vi "WSVCAP SHL Host TL I2C Read - Single Device.vi"(0 "Bytes to Read (1-4)":u8=4 min=1 max=4 step=1, 5 "Sub Address [U8]":u8=191 format="%.0x", 11 "error in":errorcluster, 12 "DUT":T2, 13 "Device":T1, 14 "Log (T)":bool=TRUE) -> (4 "Device Data":u8[](array[numeric]) format="%.0x", 15 "error out":errorcluster)   [LabVIEW 2012]
uses:
  Type Defs/WSVCAP SHL DUT Number Enum.ctl
  Type Defs/WSVCAP SHL I2C Device Enum.ctl
panel:
  out "C3:1-36 Read Data [U8]":u8[][](array[numeric]) format="%.0x"
  out "Socket Mask Set [U64]":u64[](array[numeric]) format="%012x"
  out "C2:1-36 Read Data [U8]":u8[][](array[numeric]) format="%.0x"
  out "C1:1-36 Read Data [U8]":u8[][](array[numeric]) format="%.0x"
  out "Data Headers":u8[](array[numeric])=[1, 2, 3, 4, 5, 6, 7, 8, 9, 10, 11, 12, 12, 14, 15, 16, 17, 18, 19, 20, 21, 22, 23, 24, 25, 26, 27, 28, 29, 30, 31, 32, 33, 34, 35, 36]
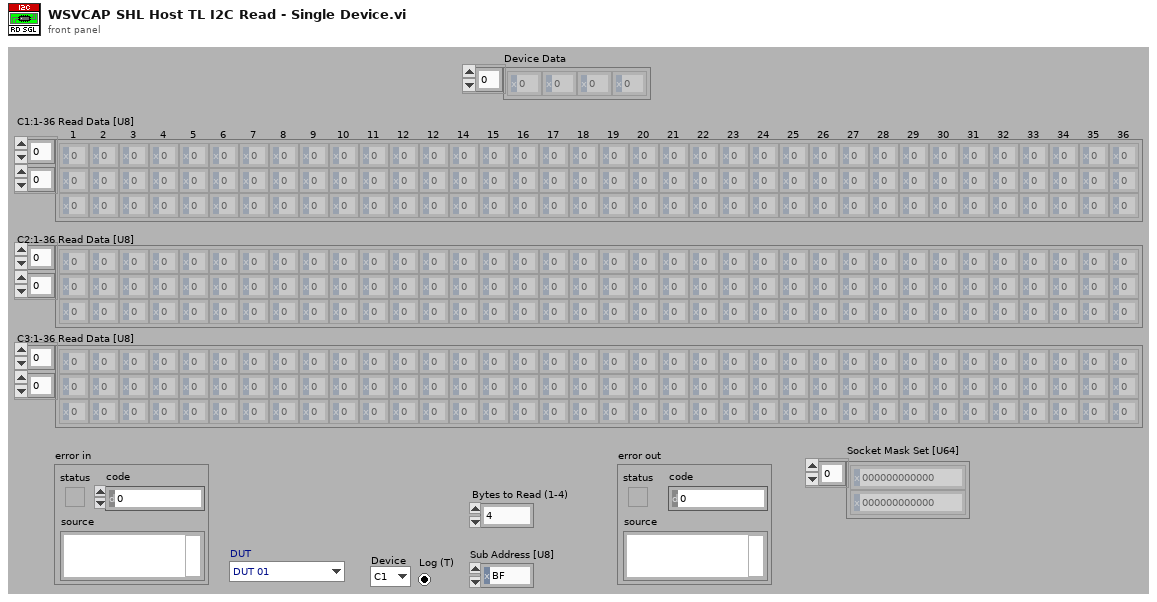
[diagram p1: front panel]
types:
  T1 = typedef "WSVCAP SHL I2C Device Enum.ctl" = enum16{"C1", "C2", "C3"}
  T2 = typedef "WSVCAP SHL DUT Number Enum.ctl" = enum16{"DUT 01", "DUT 02", "DUT 03", "DUT 04", "DUT 05", "DUT 06", "DUT 07", "DUT 08", "DUT 09", "DUT 10", "DUT 11", "DUT 12", "DUT 13", "DUT 14", "DUT 15", "DUT 16", "DUT 17", "DUT 18", "DUT 19", "DUT 20", "DUT 21", "DUT 22", "DUT 23", "DUT 24", "DUT 25", "DUT 26", "DUT 27", "DUT 28", "DUT 29", "DUT 30", "DUT 31", "DUT 32", "DUT 33", "DUT 34", "DUT 35", "DUT 36"}
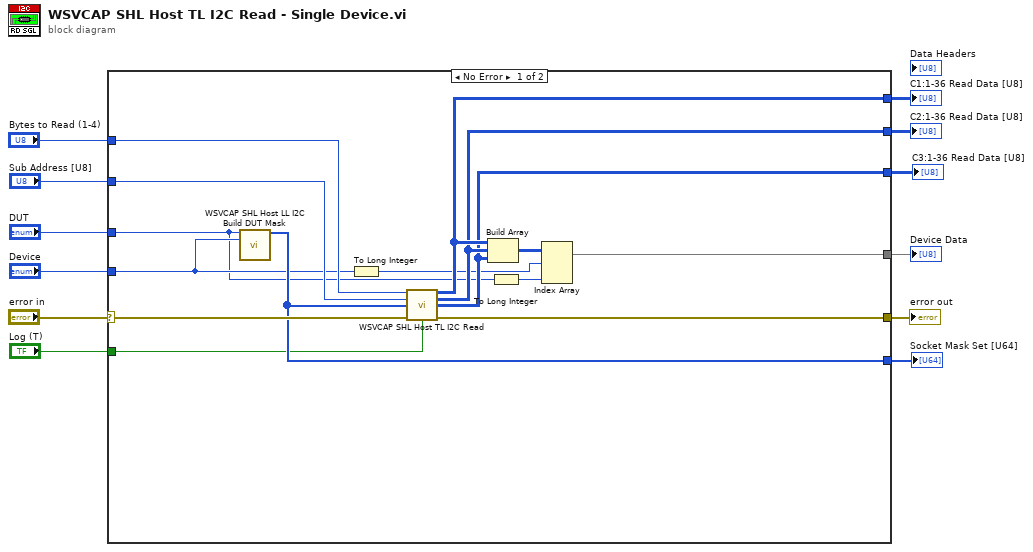
[diagram p0: block diagram]
diagram:
  n1 = case shown="No Error" "error in" {
    selector: "error in" -> [w26 w28]
    tunnel: [w27 w28] -> w12
    tunnel: "Bytes to Read (1-4)" -> [w25 _]
    tunnel: "Sub Address [U8]" -> [w24 _]
    tunnel: "DUT" -> [w13 _]
    tunnel: [w23 _] -> w7
    tunnel: "Device" -> [w15 _]
    tunnel: [w20 _] -> w5
    tunnel: [w19 _] -> w4
    tunnel: [w22 _] -> w3
    tunnel: "Log (T)" -> [w21 _]
    tunnel: [w18 _] -> w1
    frame No Error {
      n2 = call "WSVCAP SHL Host LL I2C Build DUT Mask.vi"("DUT"=w13, "Device"=w15) -> ("Socket Mask Set [U64]"=w23:u64[])  [unwired: 12 in, 1 out]
      n3 = To Long Integer(number=w15) -> (32bit integer=w14:i32)
      n4 = call "WSVCAP SHL Host TL I2C Read.vi"("Bytes to Read"=w25, "Sub Address [U8]"=w24, "Socket Mask Set [U64]"=w23, "error in"=w26, "Log (T)"=w21) -> ("C1 Read Data Out"=w20:u8[][], "C2 Read Data Out"=w19:u8[][], "C3 Read Data Out"=w18:u8[][], "error out"=w27:errorcluster)  [unwired: 7 in]
      n5 = Build Array(w20, w19, w18) -> (w17:u8[][][])
      n6 = To Long Integer(number=w13) -> (32bit integer=w16:i32)
      n7 = Index Array(array=w17, index (dim 0)=w14, index (dim 2)=w16) -> (element=w22:u8[])  [unwired: 1 in]
    }
    frame Error {
    }
  }
  "error out" <- w12
  "Socket Mask Set [U64]" <- w7
  "C1:1-36 Read Data [U8]" <- w5
  "C2:1-36 Read Data [U8]" <- w4
  "Device Data" <- w3
  "C3:1-36 Read Data [U8]" <- w1
